vi "ReadTraceQueue.vi"(8 "Error In":errorcluster, 11 "reference in":refnum<class "TraceWindow.lvclass">) -> (0 "Error Out":errorcluster, 2 "TraceQueue":refnum<queue>, 3 "reference in":refnum<class "TraceWindow.lvclass">)   [LabVIEW 2021, in "TraceWindow.lvlib" / "TraceWindow.lvclass"]
uses:
  TraceWindow.lvclass
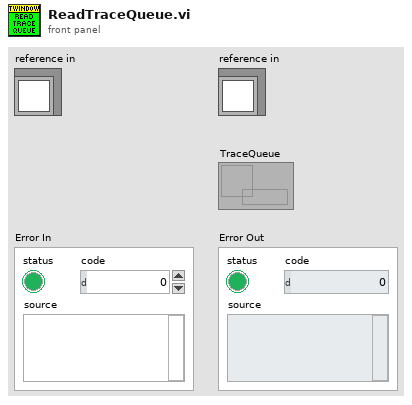
[diagram p1: front panel]
types:
  T1 = typedef "TraceWindow.lvlib/TraceWindow.lvclass/ObjectAttributes.ctl" = cluster{"Interfaces":cluster{"Dummys":refnum<class>}, "Locals":cluster{"MainGUIActive":refnum<queue>, "TraceQueue":refnum<queue>}, "Persistent":cluster{"OpenAtClosure":bool, "BufferSize":i32, "Startup":cluster{"OpenAtStartUp":bool, "OpenMinimized":bool}}}
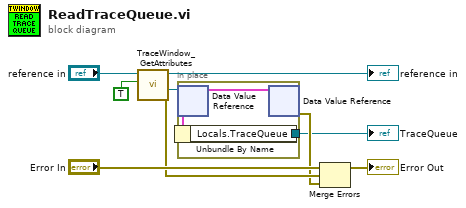
[diagram p0: block diagram]
diagram:
  n1 = call "TraceWindow_GetAttributes.vi"("OnlyGetDvrReference(False)"=TRUE, "reference in"="reference in") -> ("error out"=w6:errorcluster, "DataRef"=w3:refnum<data-value>, "reference out"=→"reference in":refnum<class "TraceWindow.lvclass">)  [unwired: 6 in, 1 out]
  n2 = in-place {
    in-place-border: [w11] -> w1
    n3 = in-place-dvr #1(w3) -> (w10:T1)  [unwired: 1 out]
    n4 = Unbundle By Name(w10) -> ("Locals.TraceQueue"=w11:refnum<queue>)
    n5 = in-place-dvr #1(w10) -> (w2:errorcluster)  [unwired: 1 out]
  }
  "TraceQueue" <- w1
  n6 = Merge Errors("Error In", w6, w2) -> (→"Error Out":errorcluster)
